vi "Send ShapePropertyChange Event.vi"(8 "error in (no error)":errorcluster, 11 "Editor Handler in":refnum<class "Image Editor Handler.lvclass">) -> (0 "error out":errorcluster, 3 "Editor Handler out":refnum<class "Image Editor Handler.lvclass">)   [LabVIEW 2017, in "LV Image Editor Framework.lvlib" / "Image Editor Handler.lvclass"]
uses:
  Image Editor Handler.lvclass
  Image Editor Handler.lvclass/Image Editor Handler.ctl
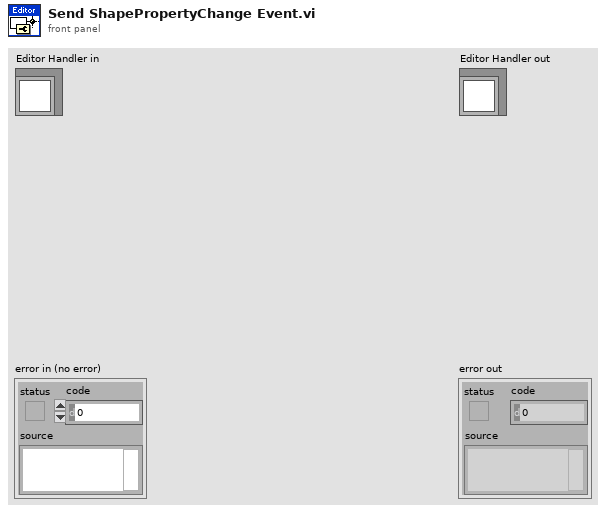
[diagram p1: front panel]
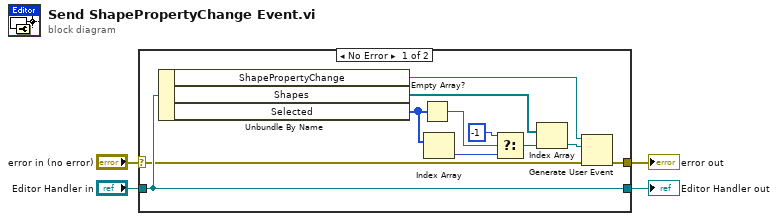
[diagram p0: block diagram]
diagram:
  n1 = case shown="No Error" "error in (no error)" {
    selector: "error in (no error)" -> [w14 w17]
    tunnel: [w13 w17] -> w3
    tunnel: [w15 w16] -> w1
    tunnel: "Editor Handler in" -> [w15 w16]
    frame No Error {
      n2 = Unbundle By Name(w15) -> ("ShapePropertyChange"=w5:refnum<user-event>, "Shapes"=w12:refnum<data-value>[], "Selected"=w9:i16[])
      n3 = Empty Array?(array=w9) -> (empty?=w10:bool)
      n4 = Index Array(array=w9) -> (element=w8:i16)  [unwired: 1 in]
      n5 = Select(t=i16 -1, s=w10, f=w8) -> (s? t:f=w6:i16)
      n6 = Index Array(array=w12, index=w6) -> (element=w11:refnum<data-value>)
      n7 = Generate User Event(user event=w5, event data cluster=w11, error in=w14) -> (error out=w13:errorcluster)  [unwired: 1 in, 1 out]
    }
    frame Error {
    }
  }
  "error out" <- w3
  "Editor Handler out" <- w1
